vi "Destroy Class.vi"(8 "error in (no error)":errorcluster, 11 "DataQueues in":refnum<class "DataQueues.lvclass">) -> (0 "error out":errorcluster, 3 "DataQueues out":refnum<class "DataQueues.lvclass">)   [LabVIEW 2017, in "DataQueues.lvclass"]
doc: "Developed by Kevin Thompson\nkevin@thompsonengineering.net\n\nCopyright 2018-2020\nThompson Engineering, LLC"
uses:
  DataQueues.lvclass
  DataQueues.lvclass/DataQueues.ctl
  Accessors/Get DataQ Dict.vi
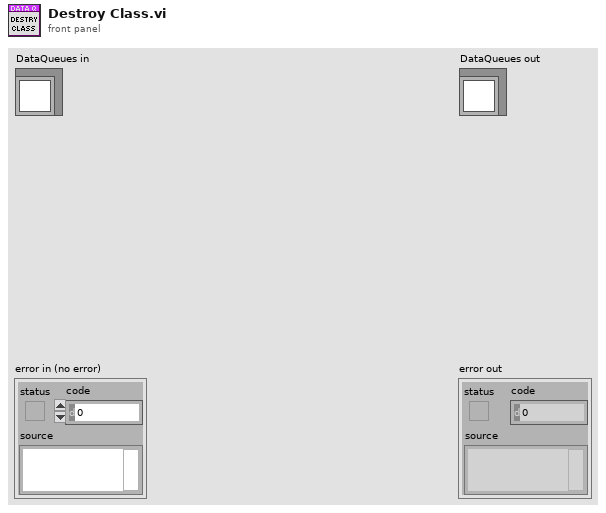
[diagram p1: front panel]
types:
  T1 = typedef "TD Dynamic CVT DVR--ref.ctl" = refnum<data-value>
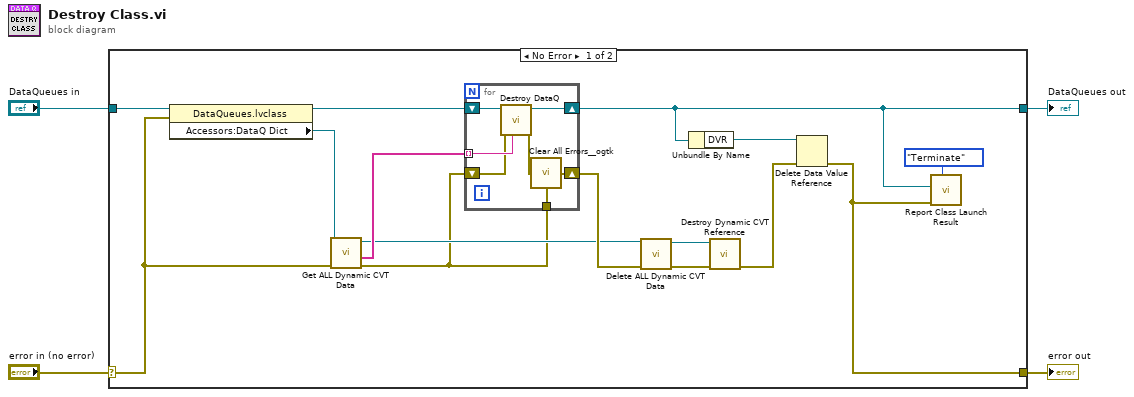
[diagram p0: block diagram]
diagram:
  n1 = case shown="No Error" "error in (no error)" {
    selector: "error in (no error)" -> [w13 w28]
    tunnel: [w6 w28] -> w3
    tunnel: [w5 w27] -> w1
    tunnel: "DataQueues in" -> [w17 w27]
    frame No Error {
      n2 = property class="DataQueues.lvclass"(reference=w17, error in=w13) -> (reference out=w15:refnum<class "DataQueues.lvclass">, "Accessors:DataQ Dict"=w16:T1)  [unwired: 1 out]
      n3 = call <vilib>:"Get ALL Dynamic CVT Data.vi"("error in (no error)"=w13, "dCVT DVR"=w16) -> ("error out"=w10:errorcluster, "NameArray"=w14:string[], "dCVT DVR out"=w11:T1)  [unwired: 6 in, 1 out]
      n4 = for {
        shift-right: [w25] -> w5
        shift-left: w15 -> [w26]
        tunnel: w14 -> [w24] mode=indexing
        shift-right: [w21] -> w12
        shift-left: w10 -> [w23]
        tunnel: w10 -> [w20]
        n5 = call "Destroy DataQ.vi"("QueueName String (optional, otherwise \"\")"=w24, "error in (no error)"=w23, "DataQueues in"=w26) -> ("error out"=w22:errorcluster, "DataQueues out"=w25:refnum<class "DataQueues.lvclass">)  [unwired: 6 in, 1 out]
        n6 = call <userlib>:"Clear All Errors__ogtk.vi"("Upsteam Error (optional)"=w20, "Error In"=w22) -> ("Error Out"=w21:errorcluster)  [unwired: 2 in]
      }
      n7 = call <vilib>:"Delete ALL Dynamic CVT Data.vi"("error in (no error)"=w12, "dCVT DVR"=w11) -> ("error out"=w9:errorcluster, "dCVT DVR out"=w19:T1)  [unwired: 8 in]
      n8 = Unbundle By Name(w5) -> ("DVR"=w18:refnum<data-value>)
      n9 = call <vilib>:"Destroy Dynamic CVT Reference.vi"("error in (no error)"=w9, "dCVT DVR"=w19) -> ("error out"=w8:errorcluster)  [unwired: 8 in, 1 out]
      n10 = Delete Data Value Reference(data value reference=w18, error in=w8) -> (error out=w6:errorcluster)  [unwired: 1 out]
      n11 = call "Report Class Launch Result.vi"("Object"=w5, "error in (no error)"=w6, "Mode (Launch)"=enum16{"Launch", "Terminate"}."Terminate") -> ()  [unwired: 7 in, 1 out]
    }
    frame Error {
    }
  }
  "error out" <- w3
  "DataQueues out" <- w1
